vi "SMU Switch Handshaking - LV code improvements - Streaming.vi"(8 "error in":errorcluster, 9 "Error Stream gRPCid":T1, 10 "gRPCid":T1, 11 "file path (use dialog)":path=path "/home/lvuser/jsontestfile.json") -> (0 "error out":errorcluster, 3 "Elapsed Time":u32)   [LabVIEW 2019]
uses:
  labview-grpc-query-server/VIs/MeasurementServer_gRPCid.ctl
  <instrlib>/niDCPower/nidcpower.llb/niDCPower Send Software Edge Trigger - Signal.ctl
  Global Operations.ctl
  labview-grpc-query-server/VIs/MeasurementServer_FourProbeRawData.ctl
  labview-grpc-query-server/VIs/MeasurementServer_ErrorOutData.ctl
  <instrlib>/niDCPower/nidcpower.llb/niDCPower Configure Software Edge Start Trigger.vi
  <instrlib>/niDCPower/nidcpower.llb/niDCPower Configure Software Edge Sequence Advance Trigger.vi
  labview-grpc-query-server/VIs/labview-grpc-measurement-server.lvlib
  SupportVIs.lvlib
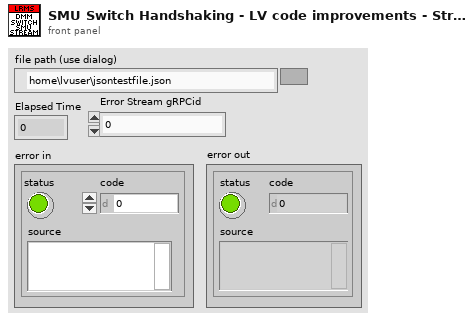
[diagram p1: front panel]
types:
  T1 = typedef "labview-grpc-measurement-server.lvlib/MeasurementServer_gRPCid.ctl" = u64
  T2 = typedef "niDCPower Send Software Edge Trigger - Signal.ctl" = i32
  T3 = typedef "JSONCluster.ctl" = cluster{"SMUResourceName":string, "SMUChannels":string, "SMUSourceMode":i32, "SMUOutputFunction":i32, "SMUSourceTransientResponse":i32, "SMUCurrent":dbl, "SMUCurrentLevelRange":dbl, "SMUMeasurementSense":i32, "SMUMeasurementApertureTime":dbl, "SMUSourceAdvancedSourceDelay":dbl, "SMUVoltage":dbl, "SMUSourceAdvancedSequenceLoopCount":i32, "SMUMeasurementAdvancedDCNoiseRejection":i32, "SMUSequenceName":string, "SMUStep1_Source_DCCurrent_CurrentLevel":i32, "SMUStep2_Measurement_ApertureTime":i32, "SMUStep3_Source_Advanced_SourceDelay":i32, "SMUSequenceNumberOfSteps":i32, "ScanList":string, "Switch1ResourceName":string, "Switch1Topology":string, "Switch1ScanList":string, "Switch2ResourceName":string, "Switch2Topology":string, "Switch2ScanList":string, "DMMResourceName":string, "DMMFunction":i32, "DMMResolution":dbl, "DMMRange":dbl, "DMMSampleCount":i32, "DMMApertureTimeUnit":i32, "DMMApertureTime":dbl, "DMMNumberOfAverages":i32, "DMMAutoZero":i32, "DMMADCCalibration":i32, "DMMSettleTime":dbl, "DMMControlAction":i32, "DMMVoltageFaultUpperLimit":dbl, "ApplicationNumberOfWeldChannels":i32}
  T4 = typedef "Global Operations.ctl" = enum16{"Get", "Set"}
  T5 = typedef "labview-grpc-measurement-server.lvlib/MeasurementServer_ErrorOutData.ctl" = cluster{"ErrorCode":i32, "ErrorMessage":string}
  T6 = typedef "labview-grpc-measurement-server.lvlib/MeasurementServer_FourProbeRawData.ctl" = cluster{"Positive Voltage":dbl, "Positive Current":dbl, "Negative Voltage":dbl, "Negative Current":dbl, "Impedance":dbl, "ErrorOutData":T5}
  T7 = typedef "niDMM Acquisition State.ctl" = enum16{"Running", "Finished with Backlog", "Finished with no Backlog", "Paused", "No acquisition in progress"}
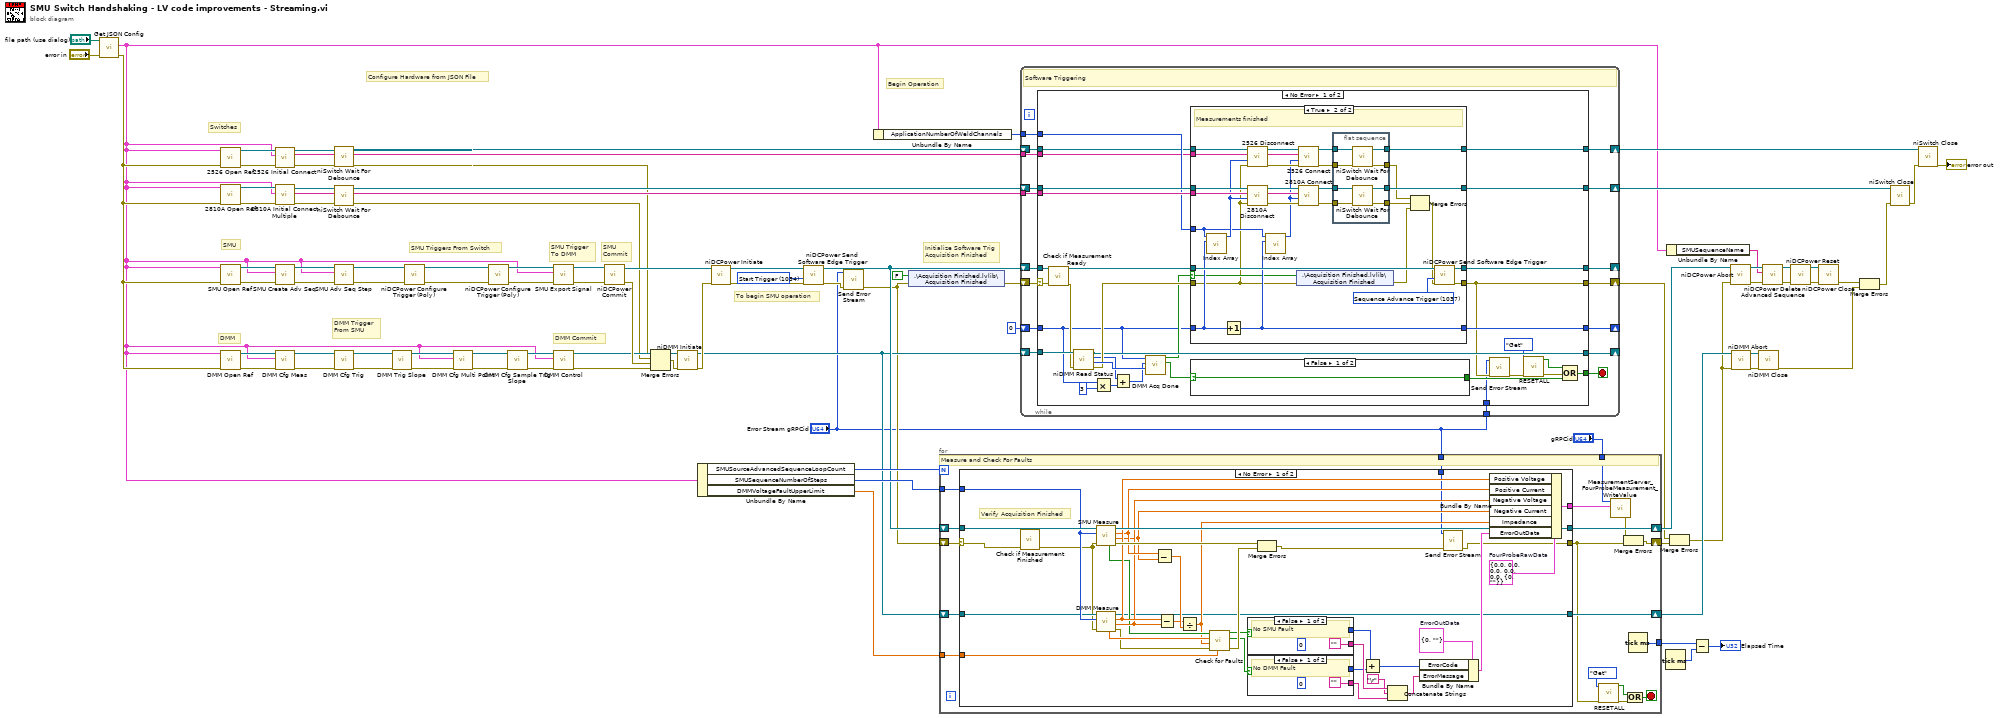
[diagram p0: block diagram]
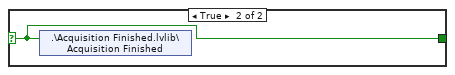
[diagram p2: hidden frame]
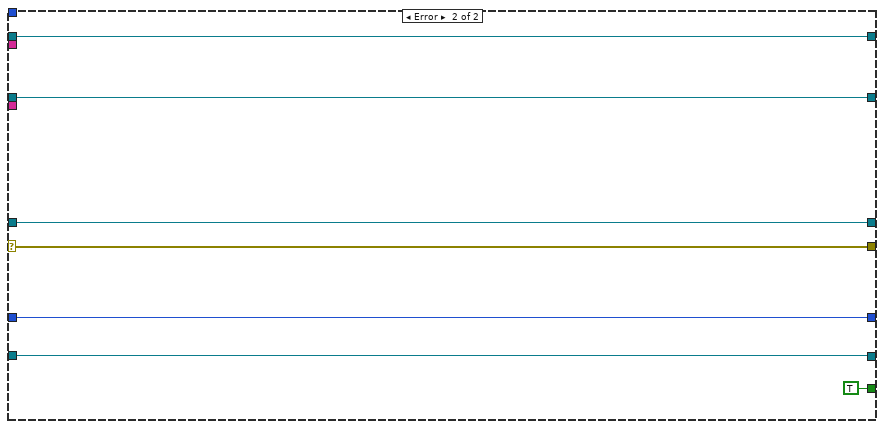
[diagram p4: hidden frame]
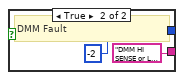
[diagram p5: hidden frame]
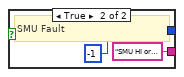
[diagram p6: hidden frame]
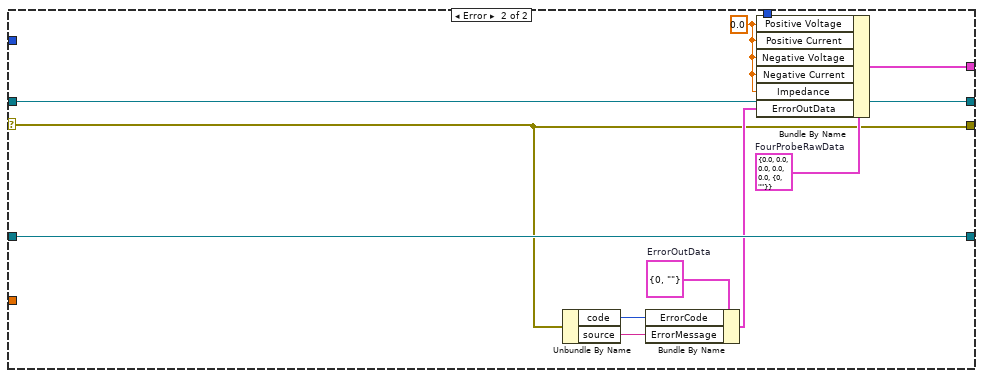
[diagram p7: hidden frame]
diagram:
  w40 = T2 1034 items=["Start Trigger"=1034, "Source Trigger"=1035, "Measure Trigger"=1036, "Sequence Advance Trigger"=1037, "Pulse Trigger"=1053] ("signal")
  # "Initialize Software Trig\nAcquisition Finished"
  # "SMU\nCommit"
  # "DMM Commit"
  # "Begin Operation"
  # "Configure Hardware from JSON File"
  # "DMM"
  # "SMU"
  # "Switches"
  # "To begin SMU operation"
  # "DMM Trigger\nFrom SMU"
  # "SMU Trigger \nTo DMM"
  # "SMU Triggers From Switch"
  n1 = call "Get JSON Config.vi"("error in (no error)"="error in", "JSON Configuration File (.json)"="file path (use dialog)") -> ("error out"=w14:errorcluster, "JSONCluster"=w10:T3)  [unwired: 6 in, 2 out]
  n2 = call "2526 Open Ref.vi"("error in"=w14, "JSONCluster"=w10) -> ("error out"=w26:errorcluster, "IVI Refnum out"=w27:refnum<k15>)  [unwired: 8 in]
  n3 = call "2810A Open Ref.vi"("error in"=w14, "JSONCluster"=w10) -> ("error out"=w33:errorcluster, "IVI Refnum out"=w34:refnum<k15>)  [unwired: 8 in]
  n4 = call "SMU Open Ref.vi"("error in (no error)"=w14, "JSONCluster"=w10) -> ("error out"=w87:errorcluster, "IVI Refnum out"=w88:refnum<k15>)  [unwired: 8 in]
  n5 = call "DMM Open Ref.vi"("error in"=w14, "JSONCluster"=w10) -> ("error out"=w60:errorcluster, "IVI Refnum out"=w59:refnum<k15>)  [unwired: 8 in]
  n6 = call "2526 Initial Connect.vi"("error in (no error)"=w26, "JSONCluster"=w10, "IVI Refnum in"=w27) -> ("error out"=w24:errorcluster, "Scan List Channels"=w20:string[], "IVI Refnum out"=w25:refnum<k15>)  [unwired: 6 in]
  n7 = call "2810A Initial Connect Multiple.vi"("error in (no error)"=w33, "JSONCluster"=w10, "IVI Refnum in"=w34) -> ("error out"=w30:errorcluster, "Scan List Channels"=w32:string[], "IVI Refnum out"=w31:refnum<k15>)  [unwired: 6 in]
  n8 = call "SMU Create Adv Seq.vi"("error in (no error)"=w87, "JSONCluster"=w10, "IVI Refnum in"=w88) -> ("error out"=w75:errorcluster, "IVI Refnum out"=w76:refnum<k15>)  [unwired: 7 in]
  n9 = call "DMM Cfg Meas.vi"("error in (no error)"=w60, "JSONCluster"=w10, "IVI Refnum in"=w59) -> ("error out"=w64:errorcluster, "IVI Refnum out"=w63:refnum<k15>)  [unwired: 7 in]
  n10 = call <instrlib>:"niSwitch Wait For Debounce.vi"("error in (no error)"=w24, "instrument handle"=w25) -> ("error out"=w22:errorcluster, "instrument handle out"=w21:refnum<k15>)  [unwired: 8 in]
  n11 = call <instrlib>:"niSwitch Wait For Debounce.vi"("error in (no error)"=w30, "instrument handle"=w31) -> ("error out"=w29:errorcluster, "instrument handle out"=w28:refnum<k15>)  [unwired: 8 in]
  n12 = call "SMU Adv Seq Step.vi"("error in (no error)"=w75, "JSONCluster"=w10, "IVI Refnum in"=w76) -> ("error out"=w73:errorcluster, "IVI Refnum out"=w74:refnum<k15>)  [unwired: 7 in]
  n13 = call "DMM Cfg Trig.vi"("error in (no error)"=w64, "IVI Refnum in"=w63) -> ("error out"=w66:errorcluster, "IVI Refnum out"=w65:refnum<k15>)  [unwired: 8 in]
  n14 = call "DMM Trig Slope.vi"("error in (no error)"=w66, "IVI Refnum in"=w65) -> ("error out"=w68:errorcluster, "IVI Refnum out"=w67:refnum<k15>)  [unwired: 8 in]
  n15 = call-poly <instrlib>:"niDCPower Configure Trigger (Poly).vi"("error in (no error)"=w73, "instrument handle"=w74) -> ("error out"=w84:errorcluster, "instrument handle out"=w85:refnum<k15>)  [unwired: 8 in]
  n16 = call "DMM Cfg Multi Point.vi"("error in (no error)"=w68, "JSONCluster"=w10, "IVI Refnum in"=w67) -> ("error out"=w70:errorcluster, "IVI Refnum out"=w69:refnum<k15>)  [unwired: 7 in]
  n17 = call-poly <instrlib>:"niDCPower Configure Trigger (Poly).vi"("error in (no error)"=w84, "instrument handle"=w85) -> ("error out"=w47:errorcluster, "instrument handle out"=w48:refnum<k15>)  [unwired: 8 in]
  n18 = call "DMM Cfg Sample Trig Slope.vi"("error in (no error)"=w70, "IVI Refnum in"=w69) -> ("error out"=w52:errorcluster, "IVI Refnum out"=w53:refnum<k15>)  [unwired: 8 in]
  n19 = call "SMU Export Signal.vi"("error in (no error)"=w47, "JSONCluster"=w10, "IVI Refnum in"=w48) -> ("error out"=w71:errorcluster, "IVI Refnum out"=w72:refnum<k15>)  [unwired: 7 in]
  n20 = call "DMM Control.vi"("error in (no error)"=w52, "JSONCluster"=w10, "IVI Refnum in"=w53) -> ("error out"=w57:errorcluster, "IVI Refnum out"=w54:refnum<k15>)  [unwired: 7 in]
  n21 = call <instrlib>:"niDCPower Commit.vi"("error in (no error)"=w71, "instrument handle"=w72) -> ("error out"=w58:errorcluster, "instrument handle out"=w55:refnum<k15>)  [unwired: 8 in]
  n22 = Merge Errors(w22, w29, w58, w57) -> (w56:errorcluster)
  n23 = call <instrlib>:"niDMM Initiate.vi"("error in (no error)"=w56, "instrument handle"=w54) -> ("error out"=w23:errorcluster, "instrument handle out"=w11:refnum<k15>)  [unwired: 8 in]
  n24 = Unbundle By Name(w10) -> ("SMUSourceAdvancedSequenceLoopCount"=w43:i32, "SMUSequenceNumberOfSteps"=w42:i32, "DMMVoltageFaultUpperLimit"=w6:dbl)
  n25 = call <instrlib>:"niDCPower Initiate.vi"("error in (no error)"=w23, "instrument handle"=w55) -> ("error out"=w35:errorcluster, "instrument handle out"=w41:refnum<k15>)  [unwired: 8 in]
  n26 = call <instrlib>:"niDCPower Send Software Edge Trigger.vi"("error in (no error)"=w35, "signal"=w40, "instrument handle"=w41) -> ("error out"=w3:errorcluster, "instrument handle out"=w12:refnum<k15>)  [unwired: 7 in]
  n27 = call "Send Error Stream.vi"("error in (no error)"=w3, "Error Stream gRPCid"="Error Stream gRPCid") -> ("error out"=w2:errorcluster)  [unwired: 9 in]
  n28 = Unbundle By Name(w10) -> ("ApplicationNumberOfWeldChannels"=w36:i32)
  n29 = shared-variable ".\\Acquisition Finished.lvlib\\Acquisition Finished"(FALSE ("Measurement Finished"), error in=w2) -> (error out=w8:errorcluster)
  n30 = for {
    N: w43 -> [_]
    tunnel: w42 -> [w101]
    shift-right: [w99] -> w13
    shift-left: w2 -> [w90]
    shift-right: [w106] -> w86
    shift-left: w12 -> [w102]
    shift-right: [w97] -> w49
    shift-left: w11 -> [w98]
    tunnel: [w105] -> w15
    tunnel: "gRPCid" -> [w104]
    tunnel: w6 -> [w96]
    tunnel: "Error Stream gRPCid" -> [w89]
    stop <- w91 stop-if-true
    # "Measure and Check For Faults"
    n31 = case shown="No Error" w90 {
      selector: w90 -> [w110 w152]
      tunnel: [w142 w160] -> w106
      tunnel: [w118 w153] -> w103
      tunnel: w102 -> [w117 w160]
      tunnel: w101 -> [w116 _]
      tunnel: w98 -> [w115 w159]
      tunnel: [w113 w159] -> w97
      tunnel: w96 -> [w111 _]
      tunnel: [w108 w152] -> w92
      tunnel: w89 -> [w107 _]
      frame No Error {
        w120 = T5 {"ErrorCode"=0, "ErrorMessage"=""}  # ErrorOutData
        w119 = T6 {"Positive Voltage"=0.0, "Positive Current"=0.0, "Negative Voltage"=0.0, "Negative Current"=0.0, "Impedance"=0.0, "ErrorOutData"={"ErrorCode"=0, "ErrorMessage"=""}}  # FourProbeRawData
        # "Verify Acquisition Finished"
        n32 = call "Check if Measurement Finished"("error in (no error)"=w110) -> ("error out"=w112:errorcluster)  [unwired: 10 in]
        n33 = call "SMU Measure.vi"("error in (no error)"=w112, "SMUSequenceNumberOfSteps"=w116, "IVI Refnum in"=w117) -> ("error out"=w141:errorcluster, "Numeric"=w134:dbl, "Numeric 2"=w136:dbl, "IVI Refnum out"=w142:refnum<k15>, "in compliance"=w123:bool[])  [unwired: 4 in]
        n34 = call "DMM Measure.vi"("error in (no error)"=w112, "SMUSequenceNumberOfSteps"=w116, "IVI Refnum in"=w115) -> ("error out"=w114:errorcluster, "Numeric"=w135:dbl, "Numeric 2"=w137:dbl, "IVI Refnum out"=w113:refnum<k15>, "Measurements"=w122:dbl[])  [unwired: 4 in]
        n35 = Subtract(x=w136, y=w134) -> (x-y=w139:dbl)
        n36 = Subtract(x=w137, y=w135) -> (x-y=w138:dbl)
        n37 = Divide(x=w138, y=w139) -> (x/y=w121:dbl)
        n38 = call "Check for Faults.vi"("DMM Voltage Fault Upper Limit"=w111, "Error In"=w114, "Resistance In"=w121, "dmm voltage measurements"=w122, "in compliance"=w123) -> ("Error Out"=w140:errorcluster, "DMM Fault"=w127:bool, "SMU Fault"=w131:bool)  [unwired: 3 in, 1 out]
        n39 = case shown="False" w131 {
          tunnel: ["" "SMU HI or LO lead disconnected\n- SMU in compliance\n- SMU Fault = True"] -> w130
          tunnel: [0 -1] -> w128
          frame False {
            # "No SMU Fault"
          }
          frame True {
            # "SMU Fault"
          }
        }
        n40 = case shown="False" w127 {
          tunnel: ["" "DMM HI SENSE or LO SENSE lead disconnected\n- DMM measures NaN, or \n- DMM overrange warning, or\n- DMM voltage > 50uV "] -> w125
          tunnel: [0 -2] -> w124
          frame False {
            # "No DMM Fault"
          }
          frame True {
            # "DMM Fault"
          }
        }
        n41 = Merge Errors(w141, w140) -> (w109:errorcluster)
        n42 = Add(x=w128, y=w124) -> (x+y=w132:i32)
        n43 = Concatenate Strings(w130, "\r", w125) -> (w129:string)
        n44 = Bundle By Name(cluster=w120, "ErrorCode"=w132, "ErrorMessage"=w129) -> (w133:T5)
        n45 = call "Send Error Stream.vi"("error in (no error)"=w109, "Error Stream gRPCid"=w107) -> ("error out"=w108:errorcluster)  [unwired: 9 in]
        n46 = Bundle By Name(cluster=w119, "Positive Voltage"=w137, "Positive Current"=w136, "Negative Voltage"=w135, "Negative Current"=w134, "Impedance"=w121, "ErrorOutData"=w133) -> (w118:T6)
      }
      frame Error {
        w151 = 0.0 ("Positive Voltage")
        w156 = T5 {"ErrorCode"=0, "ErrorMessage"=""}  # ErrorOutData
        w157 = T6 {"Positive Voltage"=0.0, "Positive Current"=0.0, "Negative Voltage"=0.0, "Negative Current"=0.0, "Impedance"=0.0, "ErrorOutData"={"ErrorCode"=0, "ErrorMessage"=""}}  # FourProbeRawData
        n47 = Unbundle By Name(w152) -> ("code"=w154:i32, "source"=w155:string)
        n48 = Bundle By Name(cluster=w156, "ErrorCode"=w154, "ErrorMessage"=w155) -> (w158:T5)
        n49 = Bundle By Name(cluster=w157, "Positive Voltage"=w151, "Positive Current"=w151, "Negative Voltage"=w151, "Negative Current"=w151, "Impedance"=w151, "ErrorOutData"=w158) -> (w153:T6)
      }
    }
    n50 = call "RESETALL.vi"("error in (no error)"=w92, "Operation"=Global_Operations."Get") -> ("error out"=w94:errorcluster, "RESETALL?"=w93:bool)  [unwired: 8 in]
    n51 = call "MeasurementServer_FourProbeMeasurement_WriteValue.vi"("gRPCid"=w104, "FourProbeRawData"=w103) -> ("error out"=w100:errorcluster)  [unwired: 8 in]
    n52 = Merge Errors(w100, w92) -> (w99:errorcluster)
    n53 = Compound Arithmetic op=OR(w93, w94) -> (w91:bool)
    n54 = Tick Count (ms)() -> (millisecond timer value=w105:u32)
  }
  n55 = while {
    shift-right: [w177] -> _
    shift-left: w12 -> [w174]
    shift-right: [w164] -> w9
    shift-left: w8 -> [w162]
    shift-right: [w175] -> w37
    shift-left: w28 -> [w176]
    shift-right: [w166] -> _
    shift-left: w11 -> [w167]
    shift-right: [w173] -> _
    shift-left: 0 ("Backlog") -> [w165]
    tunnel: w32 -> [w172]
    tunnel: w36 -> [w171]
    shift-right: [w169] -> w19
    shift-left: w21 -> [w170]
    tunnel: w20 -> [w168]
    tunnel: "Error Stream gRPCid" -> [w161]
    stop <- w163 stop-if-true
    # "Software Triggering"
    n56 = case shown="No Error" w162 {
      selector: w162 -> [w181 w256]
      tunnel: [w208 w255] -> w177
      tunnel: w176 -> [w207 w254]
      tunnel: [w206 w254] -> w175
      tunnel: w174 -> [w205 w255]
      tunnel: [w204 w257] -> w173
      tunnel: w172 -> [w203 _]
      tunnel: w171 -> [w202 _]
      tunnel: w170 -> [w201 w253]
      tunnel: [w200 w253] -> w169
      tunnel: w168 -> [w199 _]
      tunnel: w167 -> [w197 w258]
      tunnel: [w195 w258] -> w166
      tunnel: w165 -> [w190 w257]
      tunnel: [w180 w256] -> w164
      tunnel: [w182 TRUE] -> w163
      tunnel: w161 -> [w178 _]
      frame No Error {
        n57 = call "Check if Measurement Ready.vi"("error in (no error)"=w181) -> ("error out"=w193:errorcluster)  [unwired: 10 in]
        n58 = call <instrlib>:"niDMM Read Status.vi"("error in (no error)"=w193, "instrument handle"=w197) -> ("error out"=w196:errorcluster, "Acquisition State"=w198:T7, "Backlog"=w192:i32, "instrument handle out"=w195:refnum<k15>)  [unwired: 6 in]
        n59 = Multiply(x=w190, y=3) -> (x*y=w188:i32)
        n60 = Add(x=w192, y=w188) -> (x+y=w191:i32)
        n61 = call "DMM Acq Done.vi"("Acquisition State"=w198, "Backlog"=w191, "Channel Index"=w190) -> ("Finished with Backlog?"=w187:bool, "Sequence Acquision Finished?"=w194:bool)  [unwired: 7 in]
        n62 = case shown="True" w194 {
          selector: w194 -> [_ w218]
          tunnel: w196 -> [w214 w217]
          tunnel: [w215 w244] -> w208
          tunnel: [w214 w243] -> w180
          tunnel: w205 -> [w215 w240]
          tunnel: w207 -> [w213 w239]
          tunnel: [w213 w242] -> w206
          tunnel: w190 -> [w212 w223]
          tunnel: [w212 w220] -> w204
          tunnel: w203 -> [_ w236]
          tunnel: w202 -> [_ w219]
          tunnel: w201 -> [w211 w231]
          tunnel: [w211 w228] -> w200
          tunnel: w199 -> [_ w227]
          frame False {
            # "Measurements not finished yet - repeat loop"
          }
          frame True {
            w241 = T2 1037 items=["Start Trigger"=1034, "Source Trigger"=1035, "Measure Trigger"=1036, "Sequence Advance Trigger"=1037, "Pulse Trigger"=1053] ("signal")
            # "Measurements finished"
            n63 = call "Index Array.vi"("Backlog"=w223, "ApplicationNumberOfWeldChannels"=w219) -> ("Index"=w222:i32)  [unwired: 9 in]
            n64 = Increment(x=w223) -> (x+1=w220:i32)
            n65 = call "2526 Disconnect.vi"("error in (no error)"=w217, "Index"=w222, "Scan List Channels"=w227, "IVI Refnum in"=w231) -> ("error out"=w232:errorcluster, "IVI Refnum out"=w233:refnum<k15>)  [unwired: 6 in]
            n66 = call "2810A Disconnect.vi"("error in (no error)"=w217, "Index"=w222, "Scan List Channels"=w236, "IVI Refnum in"=w239) -> ("error out"=w235:errorcluster, "IVI Refnum out"=w238:refnum<k15>)  [unwired: 6 in]
            n67 = call "Index Array.vi"("Backlog"=w220, "ApplicationNumberOfWeldChannels"=w219) -> ("Index"=w221:i32)  [unwired: 9 in]
            n68 = shared-variable ".\\Acquisition Finished.lvlib\\Acquisition Finished"(w218, error in=w217) -> (error out=w216:errorcluster)
            n69 = call "2526 Connect.vi"("error in (no error)"=w232, "Index"=w221, "2525 Scan List Channels"=w227, "IVI Refnum in"=w233) -> ("error out"=w229:errorcluster, "IVI Refnum out"=w230:refnum<k15>)  [unwired: 6 in]
            n70 = call "2810A Connect.vi"("error in (no error)"=w235, "Index"=w221, "Array"=w236, "IVI Refnum in"=w238) -> ("error out"=w234:errorcluster, "IVI Refnum out"=w237:refnum<k15>)  [unwired: 6 in]
            n71 = flat-sequence {
              tunnel: [w252] -> w242
              tunnel: [w251] -> w226
              tunnel: w237 -> [w250]
              tunnel: w234 -> [w249]
              tunnel: w230 -> [w248]
              tunnel: w229 -> [w247]
              tunnel: [w246] -> w228
              tunnel: [w245] -> w225
              frame #0 {
                n72 = call <instrlib>:"niSwitch Wait For Debounce.vi"("error in (no error)"=w247, "instrument handle"=w248) -> ("error out"=w245:errorcluster, "instrument handle out"=w246:refnum<k15>)  [unwired: 8 in]
                n73 = call <instrlib>:"niSwitch Wait For Debounce.vi"("error in (no error)"=w249, "instrument handle"=w250) -> ("error out"=w251:errorcluster, "instrument handle out"=w252:refnum<k15>)  [unwired: 8 in]
              }
            }
            n74 = Merge Errors(w225, w226, w216) -> (w224:errorcluster)
            n75 = call <instrlib>:"niDCPower Send Software Edge Trigger.vi"("error in (no error)"=w224, "signal"=w241, "instrument handle"=w240) -> ("error out"=w243:errorcluster, "instrument handle out"=w244:refnum<k15>)  [unwired: 7 in]
          }
        }
        n76 = case shown="False" w187 {
          selector: w187 -> [w209 w210]
          tunnel: [w209 w210] -> w183
          frame False {
          }
          frame True {
            n77 = shared-variable ".\\Acquisition Finished.lvlib\\Acquisition Finished"(w210) -> ()  [unwired: 1 in, 1 out]
          }
        }
        n78 = call "Send Error Stream.vi"("error in (no error)"=w180, "Error Stream gRPCid"=w178) -> ("error out"=w179:errorcluster)  [unwired: 9 in]
        n79 = call "RESETALL.vi"("error in (no error)"=w179, "Operation"=Global_Operations."Get") -> ("error out"=w185:errorcluster, "RESETALL?"=w184:bool)  [unwired: 8 in]
        n80 = Compound Arithmetic op=OR(w184, w185, w183) -> (w182:bool)
      }
      frame Error {
      }
    }
  }
  n81 = Tick Count (ms)() -> (millisecond timer value=w83:u32)
  n82 = Unbundle By Name(w10) -> ("SMUSequenceName"=w16:string)
  n83 = Merge Errors(w9, w13) -> (w4:errorcluster)
  n84 = Subtract(x=w15, y=w83) -> (x-y=→"Elapsed Time":u32)
  n85 = call <instrlib>:"niDCPower Abort.vi"("error in (no error)"=w4, "instrument handle"=w86) -> ("error out"=w81:errorcluster, "instrument handle out"=w82:refnum<k15>)  [unwired: 8 in]
  n86 = call <instrlib>:"niDMM Abort.vi"("error in (no error)"=w4, "instrument handle"=w49) -> ("error out"=w62:errorcluster, "instrument handle out"=w61:refnum<k15>)  [unwired: 8 in]
  n87 = call <instrlib>:"niDMM Close.vi"("error in (no error)"=w62, "instrument handle"=w61) -> ("error out"=w51:errorcluster)  [unwired: 9 in]
  n88 = call <instrlib>:"niDCPower Delete Advanced Sequence.vi"("error in (no error)"=w81, "sequence name"=w16, "instrument handle"=w82) -> ("error out"=w80:errorcluster, "instrument handle out"=w79:refnum<k15>)  [unwired: 7 in]
  n89 = call <instrlib>:"niDCPower Reset.vi"("error in (no error)"=w80, "instrument handle"=w79) -> ("error out"=w77:errorcluster, "instrument handle out"=w78:refnum<k15>)  [unwired: 2 in, 6 out]
  n90 = call <instrlib>:"niDCPower Close.vi"("error in (no error)"=w77, "instrument handle"=w78) -> ("error out"=w50:errorcluster)  [unwired: 9 in]
  n91 = Merge Errors(w50, w51) -> (w38:errorcluster)
  n92 = call <instrlib>:"niSwitch Close.vi"("error in (no error)"=w38, "instrument handle"=w37) -> ("error out"=w18:errorcluster)  [unwired: 9 out]
  n93 = call <instrlib>:"niSwitch Close.vi"("error in (no error)"=w18, "instrument handle"=w19) -> ("error out"=→"error out":errorcluster)  [unwired: 9 out]
